vi "Import.vi"   [LabVIEW 2020, in "Custom Device Serialization.lvlib"]
uses:
  Custom Device Serialization.lvlib
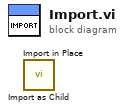
[diagram p0: block diagram]
diagram:
  n1 = call "Import as Child.vi"() -> ()  [unwired: 9 in, 3 out]
  n2 = call "Import in Place.vi"() -> ()  [unwired: 10 in, 2 out]
